vi "TIO Data Stream Subscribe Notification.vi"(4 "Notification Prefix":string, 7 "error in (no error)":errorcluster, 10 "String":string) -> (0 "error out":errorcluster)   [LabVIEW 2017]
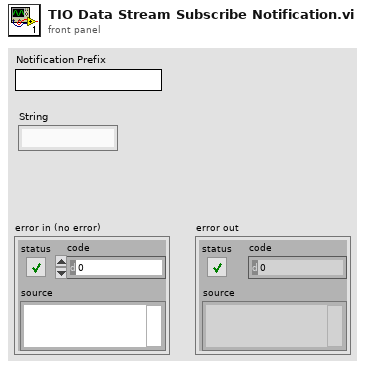
[diagram p1: front panel]
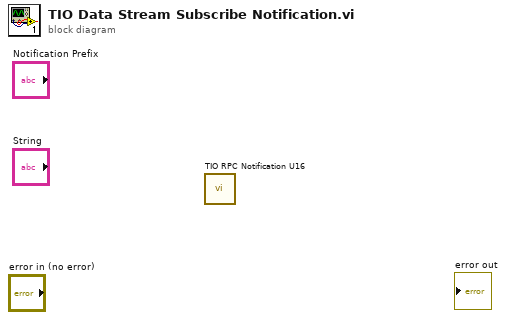
[diagram p0: block diagram]
diagram:
  n1 = call <instrlib>:"TIO RPC Notification U16.vi"() -> ()  [unwired: 8 in, 3 out]
